vi "emoji variations.vi"() -> ()   [LabVIEW 2020]
panel:
  out "Array":bool[](array[boolean])
  out "?":bool
  in  "?":bool
  out "?":bool
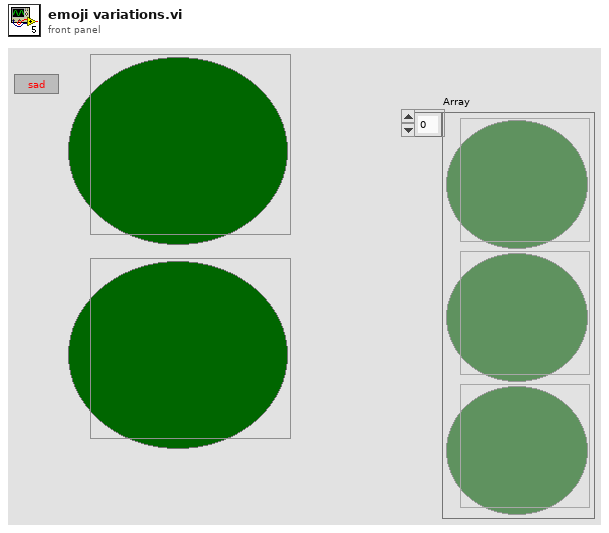
[diagram p1: front panel]
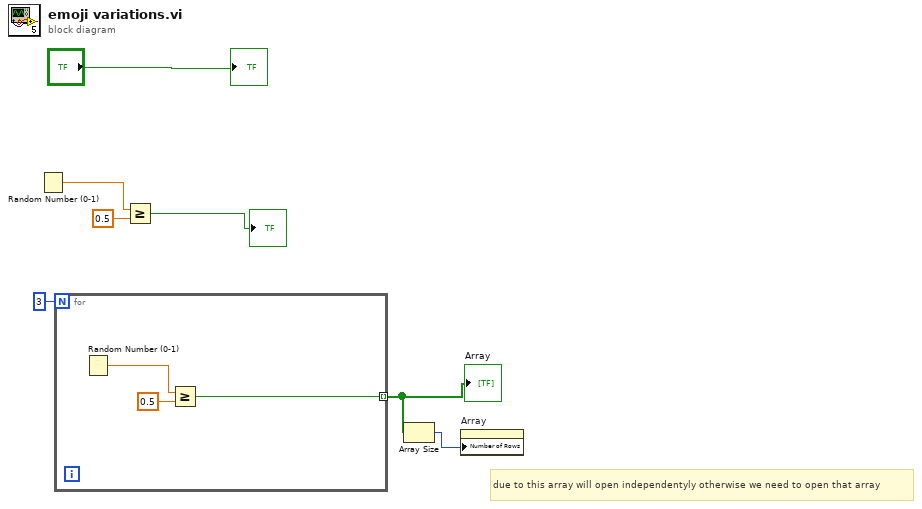
[diagram p0: block diagram]
diagram:
  # "due to this array will open independentyly otherwise we need to open that array"
  n1 = Random Number (0-1)() -> (number: 0 to 1=w5:dbl)
  n2 = for {
    N: 3 -> [_]
    tunnel: [w8] -> w2 mode=indexing
    n3 = Random Number (0-1)() -> (number: 0 to 1=w9:dbl)
    n4 = Greater Or Equal?(x=w9, y=0.5) -> (x >= y?=w8:bool)
  }
  "Array" <- w2
  n5 = Greater Or Equal?(x=w5, y=0.5) -> (x >= y?=→"?":bool)
  n6 = Array Size(array=w2) -> (size(s)=w3:i32)
  n7 = property on="Array" class="Arr (strict)"("Number of Rows"=w3) -> ()  [unwired: 2 in, 2 out]
  "?" <- "?"
